vi "Pos PID Controller.vi"(8 "error in (no error)":errorcluster, 9 "Pos Passed(deg)":dbl, 10 "Delta Motor Pos(deg)":dbl, 11 "SGDV_Ctrl_Class in":refnum<class "SGDV_Ctrl_Class.lvclass">) -> (0 "error out":errorcluster, 2 "Output Vel(deg/s)":dbl format="%.2f", 3 "SGDV_Ctrl_Class out":refnum<class "SGDV_Ctrl_Class.lvclass">)   [LabVIEW 2013, in "SGDV_Ctrl_v13_lib.lvlib" / "SGDV_Ctrl_Class.lvclass"]
uses:
  SGDV_Ctrl_Class.lvclass
  SGDV_Ctrl_Class.lvclass/SGDV_Ctrl_Class.ctl
  SGDV_Ctrl_v13_lib.lvlib
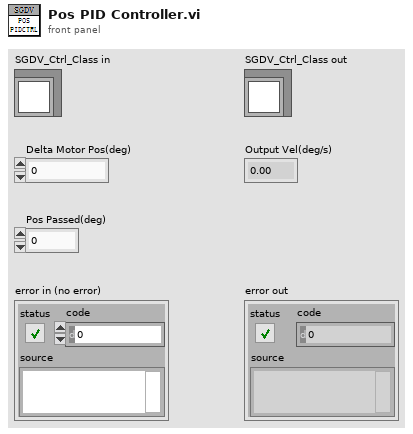
[diagram p1: front panel]
types:
  T1 = cluster{"proportional gain (Kc)":dbl, "integral time (Ti, min)":dbl, "derivative time (Td, min)":dbl}
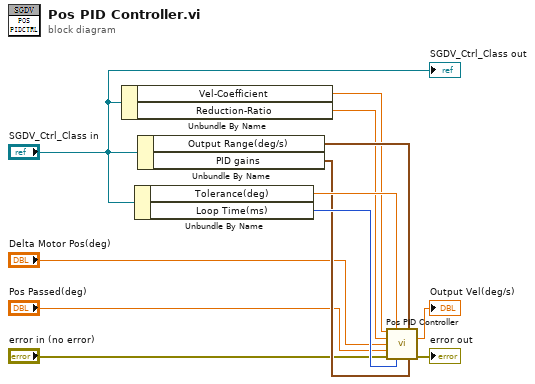
[diagram p0: block diagram]
diagram:
  n1 = Unbundle By Name("SGDV_Ctrl_Class in") -> ("Vel-Coefficient"=w7:dbl, "Reduction-Ratio"=w6:dbl)
  n2 = Unbundle By Name("SGDV_Ctrl_Class in") -> ("Tolerance(deg)"=w12:dbl, "Loop Time(ms)"=w11:u32)
  n3 = Unbundle By Name("SGDV_Ctrl_Class in") -> ("Output Range(deg/s)"=w10:cluster{"output high":dbl, "output low":dbl}, "PID gains"=w9:T1)
  n4 = call "Pos PID Controller.vi"("Vel-Coefficient"=w7, "Tolerance(deg)"=w12, "Output Range(deg/s)"=w10, "Reduction Ratio"=w6, "Delta Motor Pos(deg)"="Delta Motor Pos(deg)", "Pos Passed(deg)"="Pos Passed(deg)", "error in (no error)"="error in (no error)", "Loop Time(ms)"=w11, "PID gains"=w9) -> ("Output Vel(deg/s)"=→"Output Vel(deg/s)":dbl, "error out"=→"error out":errorcluster)  [unwired: 3 in, 2 out]
  "SGDV_Ctrl_Class out" <- "SGDV_Ctrl_Class in"
